vi "SUB_Gen3ports_MACString.vi"(5 "Port1-MAC Input":string="AABBCCDDEEFFAA") -> (0 "port3-MAC":string, 1 "port2-MAC":string, 2 "port1-MAC":string)   [LabVIEW 2011]
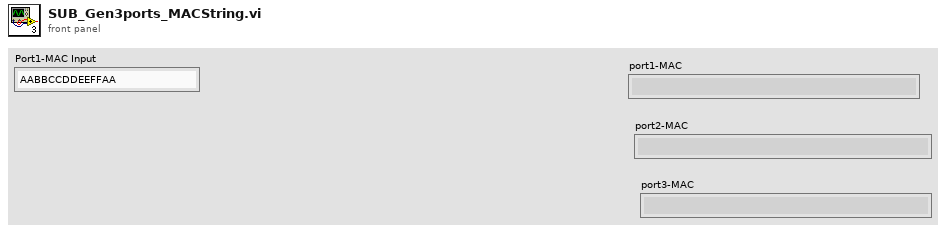
[diagram p1: front panel]
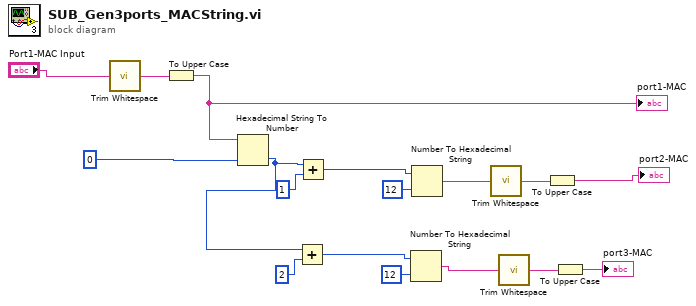
[diagram p0: block diagram]
diagram:
  n1 = call <vilib>:"Trim Whitespace.vi"("string"="Port1-MAC Input") -> ("trimmed string"=w11:string)  [unwired: 1 in]
  n2 = To Upper Case(1:w11) -> (0:w10:string)
  "port1-MAC" <- w10
  n3 = Hexadecimal String To Number(string=w10, default (0uL)=u64 0 ("default (0 U32)")) -> (number=w3:u64)  [unwired: 1 in, 1 out]
  n4 = Add(x=w3, y=u64 2) -> (x+y=w14:u64)
  n5 = Add(x=w3, y=u64 1) -> (x+y=w16:u64)
  n6 = Number To Hexadecimal String(1:i16 12 ("width (-)"), 2:w14) -> (0:w5:string)
  n7 = Number To Hexadecimal String(1:i16 12 ("width (-)"), 2:w16) -> (0:w8:string)
  n8 = call <vilib>:"Trim Whitespace.vi"("string"=w8) -> ("trimmed string"=w9:string)  [unwired: 1 in]
  n9 = call <vilib>:"Trim Whitespace.vi"("string"=w5) -> ("trimmed string"=w6:string)  [unwired: 1 in]
  n10 = To Upper Case(1:w9) -> (0:→"port2-MAC":string)
  n11 = To Upper Case(1:w6) -> (0:→"port3-MAC":string)
